vi "Global - All UI Loop Stop.vi"() -> ()   [LabVIEW 2013]
panel:
  in  "All UI Loop Stop":bool caption="全部UI循环停止"
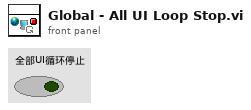
[diagram p1: front panel]
diagram:
